vi "Ball Tracking.vi"() -> ()   [LabVIEW 2013]
panel:
  in  "Min. Power":dbl=0.15 format="%#_13g"
  in  "Turn Speed":dbl
  in  "Turn Limit":dbl format="%#_13g"
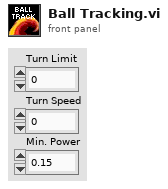
[diagram p1: front panel]
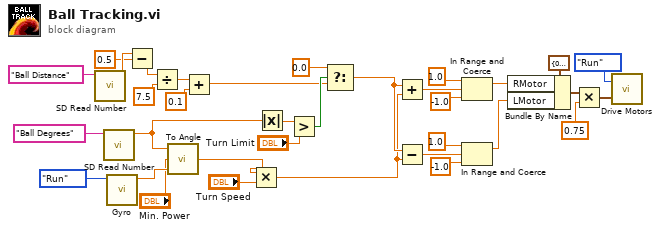
[diagram p0: block diagram]
diagram:
  n1 = call <vilib>:"SD Read Number.vi"("Name"="Ball Distance") -> ("Numeric"=w8:dbl)  [unwired: 8 in, 2 out]
  n2 = call <vilib>:"SD Read Number.vi"("Name"="Ball Degrees") -> ("Numeric"=w14:dbl)  [unwired: 8 in, 2 out]
  n3 = call "Gyro.vi"("Enum"=enum16{"Start", "Run", "End"}."Run") -> ("Angle"=w20:dbl)  [unwired: 10 in]
  n4 = Subtract(x=w8, y=0.5) -> (x-y=w6:dbl)
  n5 = Divide(x=w6, y=7.5) -> (x/y=w18:dbl)
  n6 = call "To Angle.vi"("Current Angle"=w20, "Min. Power"="Min. Power", "Destination Angle"=w14) -> ("Power Change"=w2:dbl)
  n7 = Add(x=w18, y=0.1) -> (x+y=w4:dbl)
  n8 = Multiply(x=w2, y="Turn Speed") -> (x*y=w1:dbl)
  n9 = Absolute Value(x=w14) -> (abs(x)=w13:dbl)
  n10 = Greater?(x=w13, y="Turn Limit") -> (0:w10:bool)
  n11 = Select(t=0.0, s=w10, f=w4) -> (s? t:f=w9:dbl)
  n12 = Add(x=w9, y=w1) -> (x+y=w28:dbl)
  n13 = Subtract(x=w9, y=w1) -> (x-y=w21:dbl)
  n14 = In Range and Coerce(upper limit=1.0, x=w28, lower limit=-1.0) -> (coerced(x)=w27:dbl)  [unwired: 1 out]
  n15 = In Range and Coerce(upper limit=1.0, x=w21, lower limit=-1.0) -> (coerced(x)=w22:dbl)  [unwired: 1 out]
  n16 = Bundle By Name(cluster=cluster{"RMotor":dbl, "LMotor":dbl} {"RMotor"=0.0, "LMotor"=0.0} ("Motor Powers 2"), "RMotor"=w27, "LMotor"=w22) -> (w30:cluster{"RMotor":dbl, "LMotor":dbl})
  n17 = Multiply(x=w30, y=0.75) -> (x*y=w16:cluster{"RMotor":dbl, "LMotor":dbl})
  n18 = call "Drive Motors.vi"("Motor Powers"=w16, "Enum"=enum16{"Start", "Run", "End"}."Run") -> ()
